vi "BuildCustomDashBoardData.vi"   [LabVIEW 2011]
doc: "This VI builds data and sends it back to the dashboard PC program. By default it sends back the raw values for the first analog, digital, and solenoid module. Modify it to send back the data you want to view. Consider adding higher level data to the Dashboard Datatype.ctl and to this VI. Then update the Dashboard to display the data however you like.\n\nThis software is licensed. Open the labview\\readme\\WPI Robotics Library Open Source License.txt file for more information."
uses:
  <vilib>/Rock Robotics/WPI/DriverStation/WPI_DriverStationDigitalData.ctl
  custom dash data.ctl
  subStates.ctl
  Dashboard Datatype.ctl
  DashboardEnable.ctl
  fg_typedef.ctl
  ADXL345 I2C Axis.ctl
  <vilib>/NI_Real-Time Target Support.lvlib
types:
  T1 = typedef "DashboardEnable.ctl" = cluster{"Analog Module 1":bool[], "Analog Module 2":bool[], "Digital Module 1":bool, "Digital Module 2":bool, "Solenoid Module":bool}
  T2 = typedef "Dashboard Datatype.ctl" = cluster{cluster{"AnalogModule[0]":cluster{"Channel[0]":sgl, "Channel[1]":sgl, "Channel[2]":sgl, "Channel[3]":sgl, "Channel[4]":sgl, "Channel[5]":sgl, "Channel[6]":sgl, "Channel[7]":sgl}, "AnalogModule[1]":cluster{"Channel[0]":sgl, "Channel[1]":sgl, "Channel[2]":sgl, "Channel[3]":sgl, "Channel[4]":sgl, "Channel[5]":sgl, "Channel[6]":sgl, "Channel[7]":sgl}}, cluster{"DigitalModule[0]":T3, "DigitalModule[1]":T3}, "Solenoid":u8}
  T3 = typedef "WPI_DriverStationDigitalData.ctl" = cluster{"Relay Fwd":u8, "Relay Rev":u8, "GPIO":u16, "GPIO_OE":u16, "PWM":cluster{"PWM[0]":u8, "PWM[1]":u8, "PWM[2]":u8, "PWM[3]":u8, "PWM[4]":u8, "PWM[5]":u8, "PWM[6]":u8, "PWM[7]":u8, "PWM[8]":u8, "PWM[9]":u8}}
  T4 = typedef "custom dash data.ctl" = cluster{"doubles":cluster{"Shooter Speed":dbl, "Turret Rate":dbl, "Turret Distance":dbl, "Right Distance":dbl, "Right Rate":dbl, "Left Rate":dbl, "Left Distance":dbl, "Ang. Rate":dbl, "Angle":dbl, "Shooter Bias":dbl, "Target CoM X":dbl, "Target CoM Y":dbl}, "substates":cluster{"Shooter":T5, "Upper Belts":T5, "Lower Belts":T5, "Turret ":T5, "Drive":T5}, "bools":cluster{"VLAD Balanced":bool, "Safety":bool, "Turret Limit":bool}, "Performance":cluster{"CPU Usage":dbl, "RAM Available":u32, "Vision mSPI":u32, "Main mSPI":u32}, "Target Info":cluster{"Left":i32, "Top":i32, "Right":i32, "Bottom":i32}}
  T5 = typedef "subStates.ctl" = enum16{"null", "wait", "driver control", "auto", "manual override", "autoDrive", "hold position", "rotate", "end"}
  T6 = cluster{"doubles":cluster{"Shooter Speed":dbl, "Turret Rate":dbl, "Turret Distance":dbl, "Right Distance":dbl, "Right Rate":dbl, "Left Rate":dbl, "Left Distance":dbl, "Ang, Rate":dbl, "Angle":dbl}, "substates":cluster{"Shooter":T5, "Upper Belts":T5, "Lower Belts":T5, "Turret ":T5, "Drive":T5}, "bools":cluster{"VLAD Balakced":bool, "Safety":bool}}
  T7 = typedef "fg_typedef.ctl" = enum16{"Get", "Set"}
  T8 = cluster{"AnalogModule[0]":cluster{"Channel[0]":sgl, "Channel[1]":sgl, "Channel[2]":sgl, "Channel[3]":sgl, "Channel[4]":sgl, "Channel[5]":sgl, "Channel[6]":sgl, "Channel[7]":sgl}, "AnalogModule[1]":cluster{"Channel[0]":sgl, "Channel[1]":sgl, "Channel[2]":sgl, "Channel[3]":sgl, "Channel[4]":sgl, "Channel[5]":sgl, "Channel[6]":sgl, "Channel[7]":sgl}}
  T9 = cluster{"DigitalModule[0]":T3, "DigitalModule[1]":T3}
  T10 = cluster{"Channel[0]":sgl, "Channel[1]":sgl, "Channel[2]":sgl, "Channel[3]":sgl, "Channel[4]":sgl, "Channel[5]":sgl, "Channel[6]":sgl, "Channel[7]":sgl}[]
  T11 = cluster{"Channel[0]":sgl, "Channel[1]":sgl, "Channel[2]":sgl, "Channel[3]":sgl, "Channel[4]":sgl, "Channel[5]":sgl, "Channel[6]":sgl, "Channel[7]":sgl}
  T12 = cluster{"AnalogModule[0][0]":sgl, "AnalogModule[0][1]":sgl, "AnalogModule[0][2]":sgl, "AnalogModule[0][3]":sgl, "AnalogModule[0][4]":sgl, "AnalogModule[0][5]":sgl, "AnalogModule[0][6]":sgl, "AnalogModule[0][7]":sgl}
  T13 = cluster{"[0]":cluster{"Channel[0]":sgl, "Channel[1]":sgl, "Channel[2]":sgl, "Channel[3]":sgl, "Channel[4]":sgl, "Channel[5]":sgl, "Channel[6]":sgl, "Channel[7]":sgl}, "[1]":cluster{"Channel[0]":sgl, "Channel[1]":sgl, "Channel[2]":sgl, "Channel[3]":sgl, "Channel[4]":sgl, "Channel[5]":sgl, "Channel[6]":sgl, "Channel[7]":sgl}}
  T14 = typedef "FPGA_DIODevRef.ctl" = cluster{"DevStatus":errorcluster, "Module":T15}
  T15 = typedef "FPGA_TypedefDigitalModule.ctl" = enum16{"Digital Module 1", "Digital Module 2"}
  T16 = cluster{"[0]":u8, "[1]":u8, "[2]":u8, "[3]":u8, "[4]":u8, "[5]":u8, "[6]":u8, "[7]":u8, "[8]":u8, "[9]":u8}
  T17 = typedef "FPGA_SolenoidDevRef.ctl" = cluster{"DevStatus":errorcluster, "Module":T18}
  T18 = typedef "FPGA_TypedefSolenoidModule.ctl" = enum16{"Solenoid Module 1", "Solenoid Module 2"}
  T19 = typedef "vision data.ctl" = cluster{"x":dbl, "y":dbl, "area":dbl, "width":dbl, "height":dbl}
  T20 = cluster{"Shooter Speed":dbl, "Turret Rate":dbl, "Turret Distance":dbl, "Right Distance":dbl, "Right Rate":dbl, "Left Rate":dbl, "Left Distance":dbl, "Ang. Rate":dbl, "Angle":dbl, "Shooter Bias":dbl, "Target CoM X":dbl, "Target CoM Y":dbl}
  T21 = cluster{"VLAD Balanced":bool, "Safety":bool, "Turret Limit":bool}
  T22 = cluster{"CPU Usage":dbl, "RAM Available":u32, "Vision mSPI":u32, "Main mSPI":u32}
  T23 = cluster{"Left":i32, "Top":i32, "Right":i32, "Bottom":i32}
  T24 = typedef "WPI_EncoderDevRef.ctl" = cluster{"DevStatus":errorcluster, "EncoderIndex":T25, "CounterIndex":T26, "DistancePerCount":dbl, "Decoding Type":T27}
  T25 = typedef "FPGA_EncoderIdx.ctl" = enum8{"Enc 0", "Enc 1", "Enc 2", "Enc 3", "Invalid"}
  T26 = typedef "FPGA_CounterCtrSystemIndex.ctl" = enum8{"Ctr 0", "Ctr 1", "Ctr 2", "Ctr 3", "Ctr 4", "Ctr 5", "Ctr 6", "Ctr 7", "Invalid"}
  T27 = typedef "WPI_EncoderType.ctl" = enum16{"1x", "2x", "4x"}
  T28 = typedef "ADXL345 I2C Axis.ctl" = u8
  T29 = typedef "WPI_I2CDevRef.ctl" = cluster{"DevStatus":errorcluster, "Digital Module":T15, "Device Address":u8}
  T30 = typedef "WPI_GyroDevRef.ctl" = cluster{"DevStatus":errorcluster, "Analog Module":T31, "Analog Channel":T32, "Offset":dbl, "Gain (VoltsPerDegree/Second)":dbl}
  T31 = typedef "FPGA_TypedefAnalogModule.ctl" = enum16{"Analog Module 1", "Analog Module 2"}
  T32 = typedef "FPGA_AIChannel.ctl" = enum8{"AI 1", "AI 2", "AI 3", "AI 4", "AI 5", "AI 6", "AI 7", "AI 8", "Invalid"}
  T33 = typedef "WPI_MotorControlDeviceRef.ctl" = cluster{"DeviceStatus":errorcluster, "Type":enum16{"PWM", "CAN"}, "PWM":cluster{"Digital Module":T15, "PWM Channel":T34, "DeadBand":T35}, "CAN":cluster{"Device Number":u8, "Control Mode":T36, "Semaphore":T37, "Max Vout":dbl}, "Invert":bool, "TransformRef":T38, "InvTransformRef":T38}
  T34 = typedef "FPGA_DIOPWMChannel.ctl" = enum8{"PWM 1", "PWM 2", "PWM 3", "PWM 4", "PWM 5", "PWM 6", "PWM 7", "PWM 8", "PWM 9", "PWM 10", "Invalid"}
  T35 = typedef "WPI_PWMDeadband.ctl" = cluster{"Name":string, "maxPositivePwm":i32, "minPositivePwm":i32, "centerPwm":i32, "maxNegativePwm":i32, "minNegativePwm":i32, "angularRange":u16}
  T36 = typedef "WPI_CANJaguar_ControlMode.ctl" = enum8{"Percent VBus", "Current", "Speed", "Position", "Voltage"}
  T37 = typedef "Semaphore RefNum" = refnum<k1>
  T38 = typedef "WPI_PWMTransform_ConPane.ctl" = refnum<vi>
  T39 = typedef "NI_Real-Time Target Support.lvlib/RT CPU Load.ctl" = cluster{"Total (%)":dbl, "Time Critical (%)":dbl, "Timed Structures (%)":dbl, "High (%)":dbl, "Above Normal (%)":dbl, "Normal (%)":dbl, "Background (%)":dbl, "Idle (%)":dbl, "ISR (%)":dbl}
  T40 = cluster{"VLAD Balance":bool, "Safety":bool, "Turret Limit":bool}
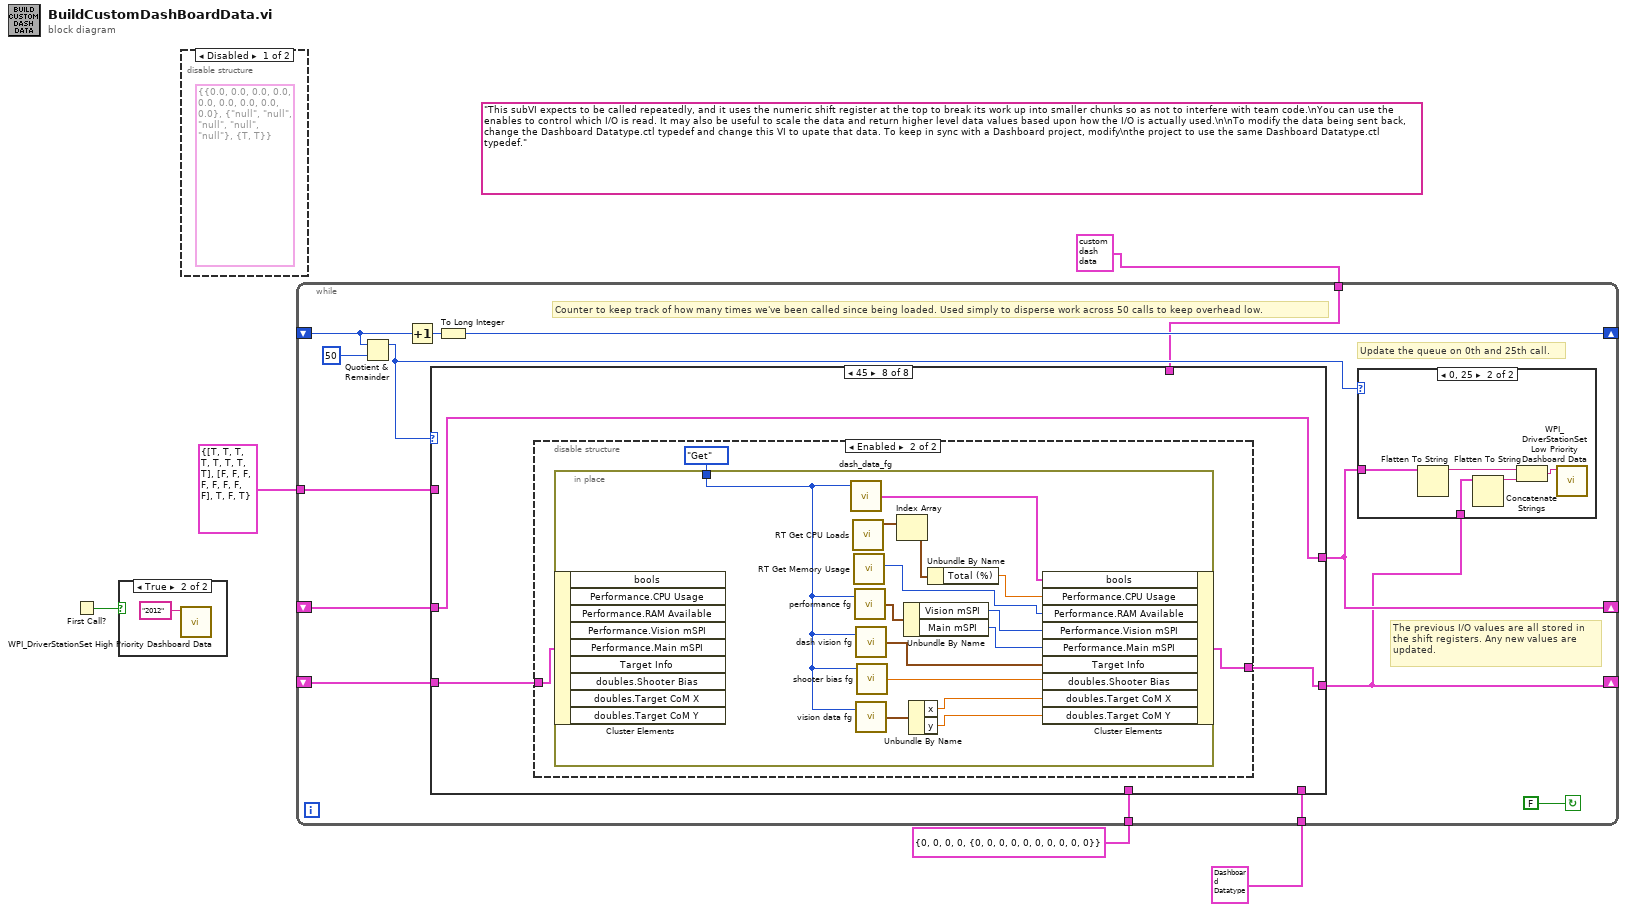
[diagram p0: block diagram]
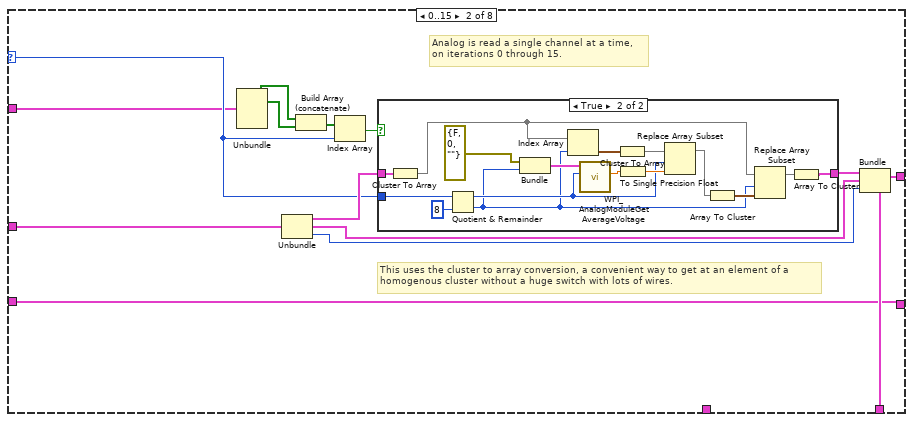
[diagram p6: hidden frame]
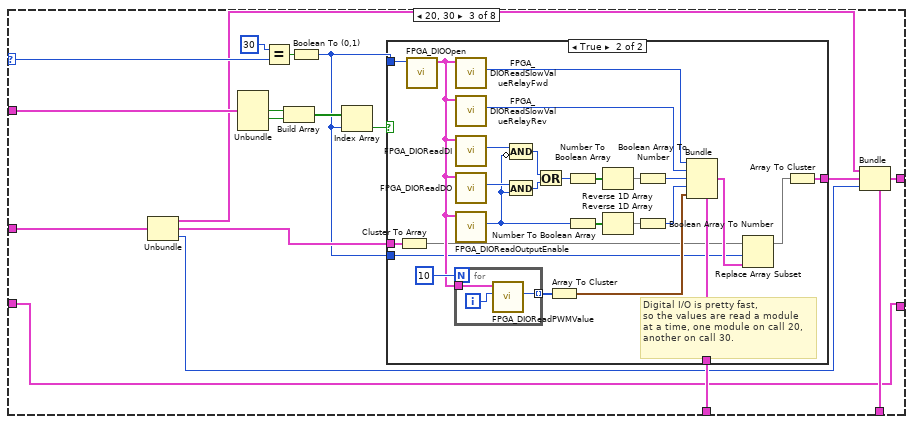
[diagram p8: hidden frame]
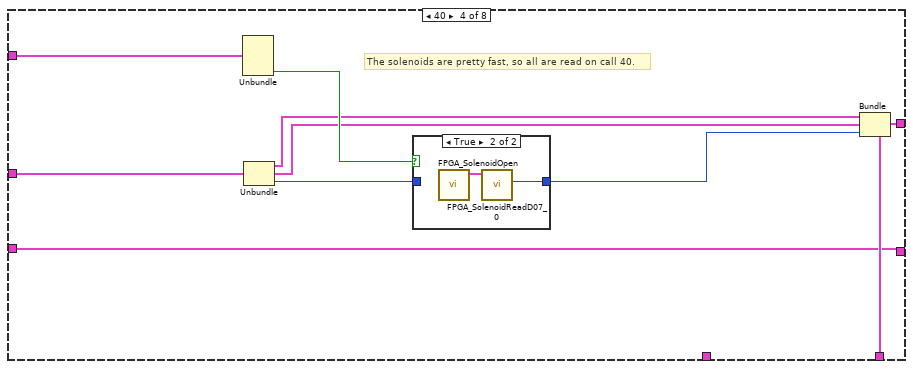
[diagram p10: hidden frame]
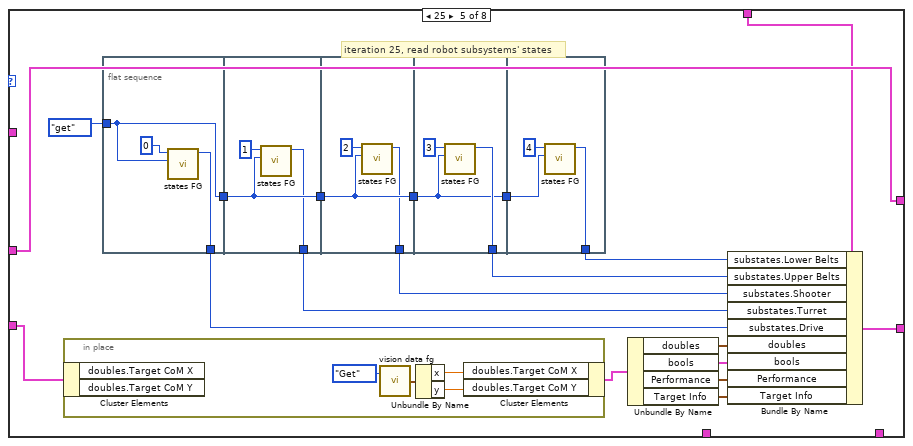
[diagram p12: hidden frame]
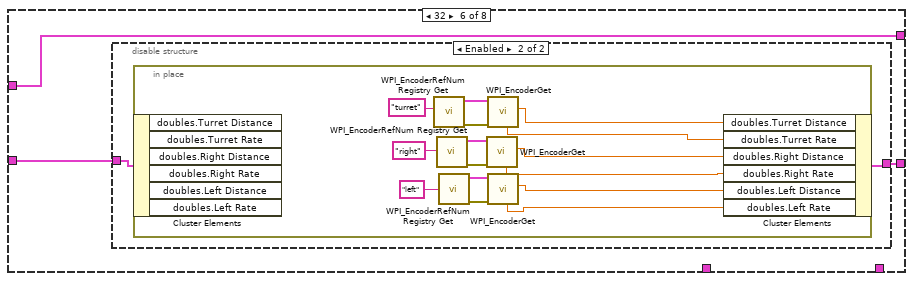
[diagram p13: hidden frame]
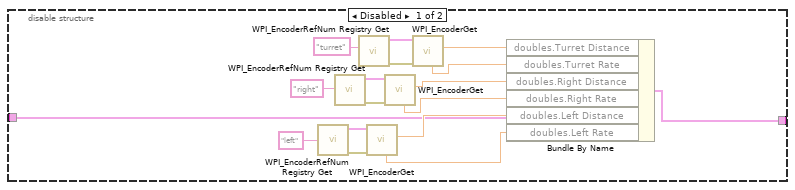
[diagram p14: hidden frame]
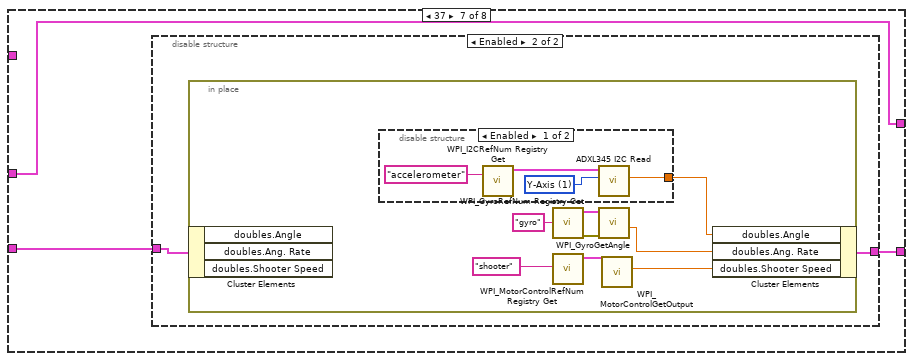
[diagram p15: hidden frame]
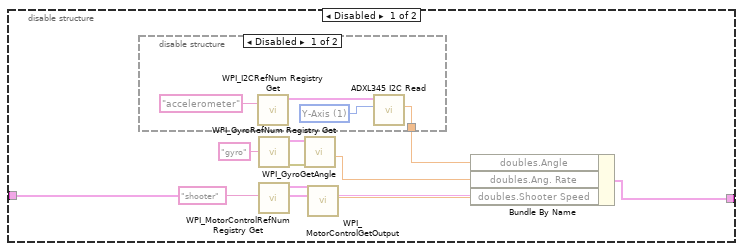
[diagram p16: hidden frame]
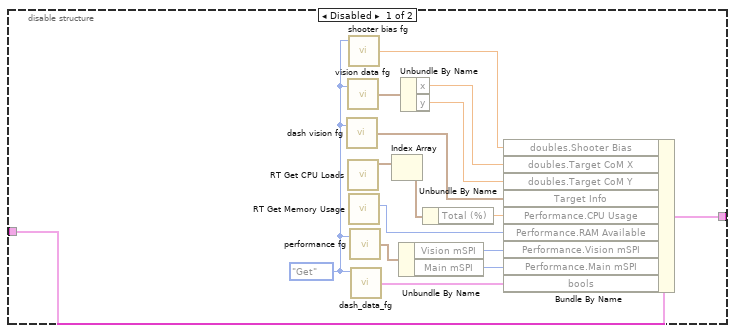
[diagram p19: hidden frame]
diagram:
  (unwired) "This subVI expects to be called repeatedly, and it uses the numeric shift register at the top to break its work up into smaller chunks so as not to interfere with team code.\nYou can use the enables to control which I/O is read. It may also be useful to scale the data and return higher level data values based upon how the I/O is actually used.\n\nTo modify the data being sent back, change the Dashboard Datatype.ctl typedef and change this VI to upate that data. To keep in sync with a Dashboard project, modify\nthe project to use the same Dashboard Datatype.ctl typedef."
  n1 = First Call?() -> (First Call?: T/F=w3:bool)
  n2 = case shown="True" w3 {
    frame False {
    }
    frame True {
      n3 = call <vilib>:"WPI_DriverStationSet High Priority Dashboard Data.vi"("User Data"="2012") -> ()  [unwired: 10 in, 1 out]
    }
  }
  n4 = disable-structure shown="Disabled" {
    frame Disabled {
      (unwired) T6 {"doubles"={"Shooter Speed"=0.0, "Turret Rate"=0.0, "Turret Distance"=0.0, "Right Distance"=0.0, "Right Rate"=0.0, "Left Rate"=0.0, "Left Distance"=0.0, "Ang, Rate"=0.0, "Angle"=0.0}, "substates"={"Shooter"=enum."null", "Upper Belts"=enum."null", "Lower Belts"=enum."null", "Turret "=enum."null", "Drive"=enum."null"}, "bools"={"VLAD Balakced"=TRUE, "Safety"=TRUE}}
    }
    frame Enabled {
    }
  }
  n5 = while {
    shift-right: [w13] -> _
    shift-left: _ -> [w15]
    shift-right: [w10] -> _
    shift-left: _ -> [w18]
    tunnel: T3 {"Relay Fwd"=0, "Relay Rev"=0, "GPIO"=0, "GPIO_OE"=0, "PWM"={"PWM[0]"=0, "PWM[1]"=0, "PWM[2]"=0, "PWM[3]"=0, "PWM[4]"=0, "PWM[5]"=0, "PWM[6]"=0, "PWM[7]"=0, "PWM[8]"=0, "PWM[9]"=0}} ("DigitalModule[1]") -> [w17]
    tunnel: T2 {{"AnalogModule[0]"={"Channel[0]"=0.0, "Channel[1]"=0.0, "Channel[2]"=0.0, "Channel[3]"=0.0, "Channel[4]"=0.0, "Channel[5]"=0.0, "Channel[6]"=0.0, "Channel[7]"=0.0}, "AnalogModule[1]"={"Channel[0]"=0.0, "Channel[1]"=0.0, "Channel[2]"=0.0, "Channel[3]"=0.0, "Channel[4]"=0.0, "Channel[5]"=0.0, "Channel[6]"=0.0, "Channel[7]"=0.0}}, {"DigitalModule[0]"={"Relay Fwd"=0, "Relay Rev"=0, "GPIO"=0, "GPIO_OE"=0, "PWM"={"PWM[0]"=0, "PWM[1]"=0, "PWM[2]"=0, "PWM[3]"=0, "PWM[4]"=0, "PWM[5]"=0, "PWM[6]"=0, "PWM[7]"=0, "PWM[8]"=0, "PWM[9]"=0}}, "DigitalModule[1]"={"Relay Fwd"=0, "Relay Rev"=0, "GPIO"=0, "GPIO_OE"=0, "PWM"={"PWM[0]"=0, "PWM[1]"=0, "PWM[2]"=0, "PWM[3]"=0, "PWM[4]"=0, "PWM[5]"=0, "PWM[6]"=0, "PWM[7]"=0, "PWM[8]"=0, "PWM[9]"=0}}}, "Solenoid"=0} ("Dashboard Data") -> [w12]
    tunnel: T1 {"Analog Module 1"=[TRUE, TRUE, TRUE, TRUE, TRUE, TRUE, TRUE, TRUE], "Analog Module 2"=[FALSE, FALSE, FALSE, FALSE, FALSE, FALSE, FALSE, FALSE], "Digital Module 1"=TRUE, "Digital Module 2"=FALSE, "Solenoid Module"=TRUE} ("Dashboard Enables") -> [w11]
    shift-right: [w7] -> _
    shift-left: _ -> [w8]
    tunnel: T4 {"doubles"={"Shooter Speed"=0.0, "Turret Rate"=0.0, "Turret Distance"=0.0, "Right Distance"=0.0, "Right Rate"=0.0, "Left Rate"=0.0, "Left Distance"=0.0, "Ang. Rate"=0.0, "Angle"=0.0, "Shooter Bias"=0.0, "Target CoM X"=0.0, "Target CoM Y"=0.0}, "substates"={"Shooter"=enum."null", "Upper Belts"=enum."null", "Lower Belts"=enum."null", "Turret "=enum."null", "Drive"=enum."null"}, "bools"={"VLAD Balanced"=FALSE, "Safety"=FALSE, "Turret Limit"=FALSE}, "Performance"={"CPU Usage"=0.0, "RAM Available"=0, "Vision mSPI"=0, "Main mSPI"=0}, "Target Info"={"Left"=0, "Top"=0, "Right"=0, "Bottom"=0}} ("Custom Dash Data") -> [w9]
    stop <- FALSE continue-if-true
    # "Counter to keep track of how many times we've been called since being loaded. Used simply to disperse work across 50 calls to keep overhead low."
    # "Update the queue on 0th and 25th call."
    # "The previous I/O values are all stored in\nthe shift registers. Any new values are\nupdated."
    n6 = Quotient & Remainder(x=w15, y=50) -> (x-y*floor(x/y)=w14:i32)  [unwired: 1 out]
    n7 = Increment(x=w15) -> (x+1=w20:i32)
    n8 = case shown="45" w14 {
      selector: w14 -> [_ w36 w72 _ _ _ _ _]
      tunnel: [w27 w32 w63 w113 w128 w159 w197 w227] -> w10
      tunnel: w18 -> [w27 w31 w65 w115 w128 w159 w197 w227]
      tunnel: w17 -> [_ _ w76 _ _ _ _ _]
      tunnel: w12 -> [_ w38 w64 w112 _ _ _ _]
      tunnel: w11 -> [_ w35 w70 w116 _ _ _ _]
      tunnel: w9 -> [_ _ _ _ w126 _ _ _]
      tunnel: [w26 w30 w61 w109 w127 w160 w196 w228] -> w7
      tunnel: w8 -> [w26 w30 w61 w109 w121 w158 w195 w226]
      frame Default {
        # "Don't update any I/O"
      }
      frame 0..15 {
        # "This uses the cluster to array conversion, a convenient way to get at an element of a\nhomogenous cluster without a huge switch with lots of wires."
        # "Analog is read a single channel at a time,\non iterations 0 through 15."
        n9 = Unbundle(w35) -> ("Analog Module 1"=w34:bool[], "Analog Module 2"=w33:bool[])  [unwired: 3 out]
        n10 = Unbundle(w31) -> (w37:T8, w29:T9, "Solenoid"=w28:u8)
        n11 = Build Array (concatenate)(w34, w33) -> (w40:bool[])
        n12 = Index Array(array=w40, index=w36) -> (element=w41:bool)
        n13 = case shown="True" w41 {
          tunnel: w36 -> [_ w49]
          tunnel: [w42 w46] -> w39
          tunnel: w37 -> [w42 w45]
          frame False {
          }
          frame True {
            n14 = Cluster To Array(cluster=w45) -> (array=w44:T10)
            n15 = Quotient & Remainder(x=w49, y=8) -> (x-y*floor(x/y)=w48:i32, floor(x/y)=w43:i32)
            n16 = Bundle("DevStatus"=errorcluster {"status"=FALSE, "code"=0, "source"=""}, w43) -> (w57:cluster{"DevStatus":errorcluster, i32})  [unwired: 1 out]
            n17 = Index Array(array=w44, index=w43) -> (element=w51:T11)
            n18 = call <vilib>:"WPI_AnalogModuleGetAverageVoltage.vi"("Channel"=w48, "AnalogModuleDevStatus"=w57) -> ("Average Voltage"=w54:dbl)  [unwired: 1 in, 8 out]
            n19 = Cluster To Array(cluster=w51) -> (array=w50:sgl[])
            n20 = To Single Precision Float(number=w54) -> (single precision float=w53:sgl)
            n21 = Replace Array Subset(array=w50, new element=w53, index=w48) -> (w52:sgl[])
            n22 = Array To Cluster(array=w52) -> (cluster=w56:T12)
            n23 = Replace Array Subset(array=w44, new element=w56, index=w43) -> (w47:T10)
            n24 = Array To Cluster(array=w47) -> (cluster=w46:T13)
          }
        }
        n25 = Bundle(cluster=w38, w39, w29, "Solenoid"=w28) -> (w32:T2)
      }
      frame 20, 30 {
        n26 = Unbundle(w65) -> (w60:T8, w67:T9, "Solenoid"=w59:u8)
        n27 = Unbundle(w70) -> ("Digital Module 1"=w69:bool, "Digital Module 2"=w68:bool)  [unwired: 3 out]
        n28 = Equal?(x=30, y=w72) -> (x = y?=w74:bool)
        n29 = Build Array(w69, w68) -> (w71:bool[])
        n30 = Boolean To (0,1)(Boolean=w74) -> (0, 1=w62:i16)
        n31 = Index Array(array=w71, index=w62) -> (element=w73:bool)
        n32 = case shown="True" w73 {
          tunnel: w76 -> [_ w85]
          tunnel: [w77 w78] -> w66
          tunnel: w62 -> [_ w83]
          tunnel: w62 -> [_ w82]
          tunnel: w67 -> [w77 w81]
          frame False {
          }
          frame True {
            # "Digital I/O is pretty fast,\nso the values are read a module\nat a time, one module on call 20,\nanother on call 30."
            n33 = Cluster To Array(cluster=w81) -> (array=w80:T3[])
            n34 = call <vilib>:"FPGA_DIOOpen.vi"("Module (Module 1)"=w83) -> ("DIODeviceRef"=w101:T14)  [unwired: 1 in, 9 out]
            n35 = for {
              N: 10 -> [_]
              tunnel: w101 -> [w106]
              tunnel: [w104] -> w102 mode=indexing
              i -> [w105]
              n36 = call <vilib>:"FPGA_DIOReadPWMValue.vi"("PWMChannel"=w105, "DIODeviceRef In"=w106) -> ("PWMValue"=w104:u8)  [unwired: 1 in, 8 out]
            }
            n37 = call <vilib>:"FPGA_DIOReadSlowValueRelayFwd.vi"("DIODeviceRef In"=w101) -> ("Relay Forward"=w94:u8)  [unwired: 1 in, 9 out]
            n38 = call <vilib>:"FPGA_DIOReadSlowValueRelayRev.vi"("DIODeviceRef In"=w101) -> ("Relay Reverse"=w95:u8)  [unwired: 1 in, 9 out]
            n39 = call <vilib>:"FPGA_DIOReadDI.vi"("DIODeviceRef In"=w101) -> ("DI"=w99:u16)  [unwired: 1 in, 9 out]
            n40 = call <vilib>:"FPGA_DIOReadDO.vi"("DIODeviceRef In"=w101) -> ("DO"=w98:u16)  [unwired: 1 in, 9 out]
            n41 = call <vilib>:"FPGA_DIOReadOutputEnable.vi"("DIODeviceRef In"=w101) -> ("OutputEnable"=w89:u16)  [unwired: 1 in, 9 out]
            n42 = And(x=w98, y=w89) -> (x .and. y?=w97:u16)
            n43 = Compound Arithmetic op=AND(w99, invert w89) -> (w96:u16)
            n44 = Or(x=w96, y=w97) -> (x .or. y?=w87:u16)
            n45 = Array To Cluster(array=w102) -> (cluster=w100:T16)
            n46 = Number To Boolean Array(number=w87) -> (Boolean array=w92:bool[])
            n47 = Number To Boolean Array(number=w89) -> (Boolean array=w91:bool[])
            n48 = Reverse 1D Array(array=w92) -> (reversed array=w93:bool[])
            n49 = Reverse 1D Array(array=w91) -> (reversed array=w90:bool[])
            n50 = Boolean Array To Number(Boolean array=w93) -> (number=w86:u32)
            n51 = Boolean Array To Number(Boolean array=w90) -> (number=w88:u32)
            n52 = Bundle(cluster=w85, "Relay Fwd"=w94, "Relay Rev"=w95, "GPIO"=w86, "GPIO_OE"=w88, "PWM"=w100) -> (w84:T3)
            n53 = Replace Array Subset(array=w80, new element=w84, index=w82) -> (w79:T3[])
            n54 = Array To Cluster(array=w79) -> (cluster=w78:cluster{"[0]":T3, "[1]":T3})
          }
        }
        n55 = Bundle(cluster=w64, w60, w66, "Solenoid"=w59) -> (w63:T2)
      }
      frame 40 {
        # "The solenoids are pretty fast, so all are read on call 40."
        n56 = Unbundle(w116) -> ("Solenoid Module"=w110:bool)  [unwired: 4 out]
        n57 = Unbundle(w115) -> (w108:T8, w107:T9, "Solenoid"=w114:u8)
        n58 = case shown="True" w110 {
          tunnel: [w117 w118] -> w111
          tunnel: w114 -> [w117 _]
          frame False {
          }
          frame True {
            n59 = call <vilib>:"FPGA_SolenoidOpen.vi"() -> ("SolenoidDevRef"=w119:T17)  [unwired: 2 in, 9 out]
            n60 = call <vilib>:"FPGA_SolenoidReadD07_0.vi"("SolenoidDevRef"=w119) -> ("DO7:0"=w118:u8)  [unwired: 1 in, 9 out]
          }
        }
        n61 = Bundle(cluster=w112, w108, w107, "Solenoid"=w111) -> (w113:T2)
      }
      frame 25 {
        # "iteration 25, read robot subsystems' states"
        n62 = in-place {
          n63 = in-place-cluster #1(w121) -> ()  [unwired: 2 out]
          n64 = call "vision data fg.vi"("Menu"=fg_typedef."Get") -> ("Data Output"=w141:T19)  [unwired: 1 in]
          n65 = Unbundle By Name(w141) -> ("x"=w140:dbl, "y"=w139:dbl)
          n66 = in-place-cluster #1("doubles.Target CoM X"=w140, "doubles.Target CoM Y"=w139) -> (w120:T4)
        }
        n67 = flat-sequence {
          tunnel: enum16{"set", "get"}."get" ("menu (get)") -> [w145]
          tunnel: [w145] -> w135
          tunnel: [w143] -> w129
          tunnel: [w148] -> w136
          tunnel: w135 -> [w148]
          tunnel: [w146] -> w130
          tunnel: [w151] -> w137
          tunnel: w136 -> [w151]
          tunnel: [w149] -> w131
          tunnel: w137 -> [w152]
          tunnel: [w153] -> w132
          tunnel: [w152] -> w134
          tunnel: w134 -> [w156]
          tunnel: [w155] -> w133
          frame #0 {
            n68 = call "states FG.vi"("menu (get)"=w145, "Loop ID"=0) -> ("subState out"=w143:T5)  [unwired: 6 in, 3 out]
          }
          frame #1 {
            n69 = call "states FG.vi"("menu (get)"=w148, "Loop ID"=1) -> ("subState out"=w146:T5)  [unwired: 6 in, 3 out]
          }
          frame #2 {
            n70 = call "states FG.vi"("menu (get)"=w151, "Loop ID"=2) -> ("subState out"=w149:T5)  [unwired: 6 in, 3 out]
          }
          frame #3 {
            n71 = call "states FG.vi"("menu (get)"=w152, "Loop ID"=3) -> ("subState out"=w153:T5)  [unwired: 6 in, 3 out]
          }
          frame #4 {
            n72 = call "states FG.vi"("menu (get)"=w156, "Loop ID"=4) -> ("subState out"=w155:T5)  [unwired: 6 in, 3 out]
          }
        }
        n73 = Unbundle By Name(w120) -> ("doubles"=w125:T20, "bools"=w124:T21, "Performance"=w123:T22, "Target Info"=w122:T23)
        n74 = Bundle By Name(cluster=w126, "substates.Lower Belts"=w133, "substates.Upper Belts"=w132, "substates.Shooter"=w131, "substates.Turret"=w130, "substates.Drive"=w129, "doubles"=w125, "bools"=w124, "Performance"=w123, "Target Info"=w122) -> (w127:T4)
      }
      frame 32 {
        n75 = disable-structure shown="Enabled" {
          disable-tunnel: [w177 w178] -> w160
          disable-tunnel: w158 -> [w161 w179]
          frame Disabled {
            n76 = call <vilib>:"WPI_EncoderRefNum Registry Get.vi"("refnum name"="left") -> ("error out"=w173:errorcluster, "EncoderDevRef"=w172:T24)  [unwired: 9 in]
            n77 = call <vilib>:"WPI_EncoderRefNum Registry Get.vi"("refnum name"="right") -> ("error out"=w171:errorcluster, "EncoderDevRef"=w170:T24)  [unwired: 9 in]
            n78 = call <vilib>:"WPI_EncoderRefNum Registry Get.vi"("refnum name"="turret") -> ("error out"=w169:errorcluster, "EncoderDevRef"=w168:T24)  [unwired: 9 in]
            n79 = call <vilib>:"WPI_EncoderGet.vi"("error in (no error)"=w173, "EncoderDevRef"=w172) -> ("Distance"=w163:dbl, "Rate"=w162:dbl)  [unwired: 4 in, 4 out]
            n80 = call <vilib>:"WPI_EncoderGet.vi"("error in (no error)"=w171, "EncoderDevRef"=w170) -> ("Distance"=w165:dbl, "Rate"=w164:dbl)  [unwired: 4 in, 4 out]
            n81 = call <vilib>:"WPI_EncoderGet.vi"("error in (no error)"=w169, "EncoderDevRef"=w168) -> ("Distance"=w167:dbl, "Rate"=w166:dbl)  [unwired: 4 in, 4 out]
            n82 = Bundle By Name(cluster=w161, "doubles.Turret Distance"=w167, "doubles.Turret Rate"=w166, "doubles.Right Distance"=w165, "doubles.Right Rate"=w164, "doubles.Left Distance"=w163, "doubles.Left Rate"=w162) -> (w177:T4)
          }
          frame Enabled {
            n83 = in-place {
              n84 = in-place-cluster #2(w179) -> ()  [unwired: 6 out]
              n85 = call <vilib>:"WPI_EncoderRefNum Registry Get.vi"("refnum name"="turret") -> ("error out"=w187:errorcluster, "EncoderDevRef"=w186:T24)  [unwired: 9 in]
              n86 = call <vilib>:"WPI_EncoderRefNum Registry Get.vi"("refnum name"="right") -> ("error out"=w189:errorcluster, "EncoderDevRef"=w188:T24)  [unwired: 9 in]
              n87 = call <vilib>:"WPI_EncoderRefNum Registry Get.vi"("refnum name"="left") -> ("error out"=w191:errorcluster, "EncoderDevRef"=w190:T24)  [unwired: 9 in]
              n88 = call <vilib>:"WPI_EncoderGet.vi"("error in (no error)"=w189, "EncoderDevRef"=w188) -> ("Distance"=w183:dbl, "Rate"=w182:dbl)  [unwired: 4 in, 4 out]
              n89 = call <vilib>:"WPI_EncoderGet.vi"("error in (no error)"=w187, "EncoderDevRef"=w186) -> ("Distance"=w185:dbl, "Rate"=w184:dbl)  [unwired: 4 in, 4 out]
              n90 = call <vilib>:"WPI_EncoderGet.vi"("error in (no error)"=w191, "EncoderDevRef"=w190) -> ("Distance"=w181:dbl, "Rate"=w180:dbl)  [unwired: 4 in, 4 out]
              n91 = in-place-cluster #2("doubles.Turret Distance"=w185, "doubles.Turret Rate"=w184, "doubles.Right Distance"=w183, "doubles.Right Rate"=w182, "doubles.Left Distance"=w181, "doubles.Left Rate"=w180) -> (w178:T4)
            }
          }
        }
      }
      frame 37 {
        n92 = disable-structure shown="Enabled" {
          disable-tunnel: [w207 w212] -> w196
          disable-tunnel: w195 -> [w198 w213]
          frame Disabled {
            n93 = disable-structure shown="Disabled" {
              disable-tunnel: [w208 _] -> w202
              frame Disabled {
                w209 = T28 1 items=["X-Axis", "Y-Axis", "Z-Axis"] ("Axis")
                n94 = call <vilib>:"WPI_I2CRefNum Registry Get.vi"("refnum name"="accelerometer") -> ("I2CDevRef"=w210:T29)  [unwired: 9 in, 1 out]
                n95 = call "ADXL345 I2C Read.vi"("Axis"=w209, "I2CDevRef"=w210) -> ("Acceleration"=w208:dbl)  [unwired: 7 in, 2 out]
              }
              frame Enabled {
              }
            }
            n96 = call <vilib>:"WPI_GyroRefNum Registry Get.vi"("refnum name"="gyro") -> ("error out"=w201:errorcluster, "GyroDevRef"=w200:T30)  [unwired: 9 in]
            n97 = call <vilib>:"WPI_MotorControlRefNum Registry Get.vi"("refnum name"="shooter") -> ("MotorControlDevRef"=w205:T33)  [unwired: 9 in, 1 out]
            n98 = call <vilib>:"WPI_GyroGetAngle.vi"("error in (no error)"=w201, "GyroDevRef"=w200) -> ("Angular Rate"=w199:dbl)  [unwired: 6 in, 3 out]
            n99 = call <vilib>:"WPI_MotorControlGetOutput.vi"("MotorControlDevRef"=w205) -> ("Output"=w204:dbl)  [unwired: 8 in, 2 out]
            n100 = Bundle By Name(cluster=w198, "doubles.Angle"=w202, "doubles.Ang. Rate"=w199, "doubles.Shooter Speed"=w204) -> (w207:T4)
          }
          frame Enabled {
            n101 = in-place {
              n102 = in-place-cluster #3(w213) -> ()  [unwired: 3 out]
              n103 = disable-structure shown="Enabled" {
                disable-tunnel: [w222 _] -> w214
                frame Enabled {
                  w225 = T28 1 items=["X-Axis", "Y-Axis", "Z-Axis"] ("Axis")
                  n104 = call <vilib>:"WPI_I2CRefNum Registry Get.vi"("refnum name"="accelerometer") -> ("I2CDevRef"=w224:T29)  [unwired: 9 in, 1 out]
                  n105 = call "ADXL345 I2C Read.vi"("Axis"=w225, "I2CDevRef"=w224) -> ("Acceleration"=w222:dbl)  [unwired: 7 in, 2 out]
                }
                frame Disabled {
                }
              }
              n106 = call <vilib>:"WPI_GyroRefNum Registry Get.vi"("refnum name"="gyro") -> ("error out"=w220:errorcluster, "GyroDevRef"=w221:T30)  [unwired: 9 in]
              n107 = call <vilib>:"WPI_MotorControlRefNum Registry Get.vi"("refnum name"="shooter") -> ("MotorControlDevRef"=w218:T33)  [unwired: 9 in, 1 out]
              n108 = call <vilib>:"WPI_GyroGetAngle.vi"("error in (no error)"=w220, "GyroDevRef"=w221) -> ("Angular Rate"=w215:dbl)  [unwired: 6 in, 3 out]
              n109 = call <vilib>:"WPI_MotorControlGetOutput.vi"("MotorControlDevRef"=w218) -> ("Output"=w216:dbl)  [unwired: 8 in, 2 out]
              n110 = in-place-cluster #3("doubles.Angle"=w214, "doubles.Ang. Rate"=w215, "doubles.Shooter Speed"=w216) -> (w212:T4)
            }
          }
        }
      }
      frame 45 {
        n111 = disable-structure shown="Enabled" {
          disable-tunnel: [w244 w245] -> w228
          disable-tunnel: w226 -> [w229 w247]
          frame Disabled {
            w231 = fg_typedef."Get" ("Menu (Get)")
            n112 = call "dash vision fg.vi"("Menu"=w231) -> ("Output"=w235:T23)  [unwired: 1 in]
            n113 = call "vision data fg.vi"("Menu"=w231) -> ("Data Output"=w234:T19)  [unwired: 1 in]
            n114 = call <vilib>:"RT Get CPU Loads.vi"() -> ("CPU loads"=w238:T39[])  [unwired: 10 in, 1 out]
            n115 = call "shooter bias fg.vi"("Menu"=w231) -> ("output"=w230:dbl)  [unwired: 2 in]
            n116 = call <vilib>:"RT Get Memory Usage.vi"() -> ("available (bytes)"=w239:u32)  [unwired: 8 in, 3 out]
            n117 = call "performance fg.vi"("Menu"=w231) -> ("Output"=w242:cluster{"Vision mSPI":u32, "Main mSPI":u32})  [unwired: 1 in]
            n118 = call "dash_data_fg.vi"("Menu (Get)"=w231) -> ("Output"=w243:T40)  [unwired: 2 in]
            n119 = Index Array(array=w238) -> (element=w237:T39)  [unwired: 1 in]
            n120 = Unbundle By Name(w242) -> ("Vision mSPI"=w240:u32, "Main mSPI"=w241:u32)
            n121 = Unbundle By Name(w234) -> ("x"=w233:dbl, "y"=w232:dbl)
            n122 = Unbundle By Name(w237) -> ("Total (%)"=w236:dbl)
            n123 = Bundle By Name(cluster=w229, "doubles.Shooter Bias"=w230, "doubles.Target CoM X"=w233, "doubles.Target CoM Y"=w232, "Target Info"=w235, "Performance.CPU Usage"=w236, "Performance.RAM Available"=w239, "Performance.Vision mSPI"=w240, "Performance.Main mSPI"=w241, "bools"=w243) -> (w244:T4)
          }
          frame Enabled {
            n124 = in-place {
              in-place-border: fg_typedef."Get" ("Menu (Get)") -> [w248]
              n125 = in-place-cluster #4(w247) -> ()  [unwired: 9 out]
              n126 = call "dash_data_fg.vi"("Menu (Get)"=w248) -> ("Output"=w250:T40)  [unwired: 2 in]
              n127 = call <vilib>:"RT Get CPU Loads.vi"() -> ("CPU loads"=w255:T39[])  [unwired: 10 in, 1 out]
              n128 = call <vilib>:"RT Get Memory Usage.vi"() -> ("available (bytes)"=w253:u32)  [unwired: 8 in, 3 out]
              n129 = call "performance fg.vi"("Menu"=w248) -> ("Output"=w249:cluster{"Vision mSPI":u32, "Main mSPI":u32})  [unwired: 1 in]
              n130 = call "dash vision fg.vi"("Menu"=w248) -> ("Output"=w257:T23)  [unwired: 1 in]
              n131 = call "vision data fg.vi"("Menu"=w248) -> ("Data Output"=w261:T19)  [unwired: 1 in]
              n132 = call "shooter bias fg.vi"("Menu"=w248) -> ("output"=w258:dbl)  [unwired: 2 in]
              n133 = Index Array(array=w255) -> (element=w256:T39)  [unwired: 1 in]
              n134 = Unbundle By Name(w249) -> ("Vision mSPI"=w252:u32, "Main mSPI"=w251:u32)
              n135 = Unbundle By Name(w261) -> ("x"=w259:dbl, "y"=w260:dbl)
              n136 = Unbundle By Name(w256) -> ("Total (%)"=w254:dbl)
              n137 = in-place-cluster #4("bools"=w250, "Performance.CPU Usage"=w254, "Performance.RAM Available"=w253, "Performance.Vision mSPI"=w252, "Performance.Main mSPI"=w251, "Target Info"=w257, "doubles.Shooter Bias"=w258, "doubles.Target CoM X"=w259, "doubles.Target CoM Y"=w260) -> (w245:T4)
            }
          }
        }
      }
    }
    n138 = To Long Integer(number=w20) -> (32bit integer=w13:i32)
    n139 = case shown="0, 25" w14 {
      tunnel: w10 -> [_ w25]
      tunnel: w7 -> [_ w23]
      frame Default {
      }
      frame 0, 25 {
        n140 = Flatten To String(anything=w25) -> (data string=w24:string)  [unwired: 1 in, 4 out]
        n141 = Flatten To String(anything=w23) -> (data string=w21:string)  [unwired: 1 in, 4 out]
        n142 = Concatenate Strings(w24, w21) -> (w22:string)
        n143 = call <vilib>:"WPI_DriverStationSet Low Priority Dashboard Data.vi"("User Data"=w22) -> ()  [unwired: 1 in, 10 out]
      }
    }
  }
